vi "convertFromFPGA.vi"(0 "Modbus in":refnum<class "Modbus.lvclass">, 5 "Data":u16[](array[numeric]), 7 "StartIndex":i32, 9 "StopIndex":i32, 11 "error in (no error)":errorcluster, 12 "Timestamp":u64) -> (4 "Modbus out":refnum<class "Modbus.lvclass">, 6 "RxFrame":T1 {"Data" format="%02x"}, 15 "error out":errorcluster)   [LabVIEW 2016, in "RTModbusFPGA.lvlib" / "Modbus.lvclass"]
uses:
  Modbus.lvclass
  DataTypes/RxFrame.ctl
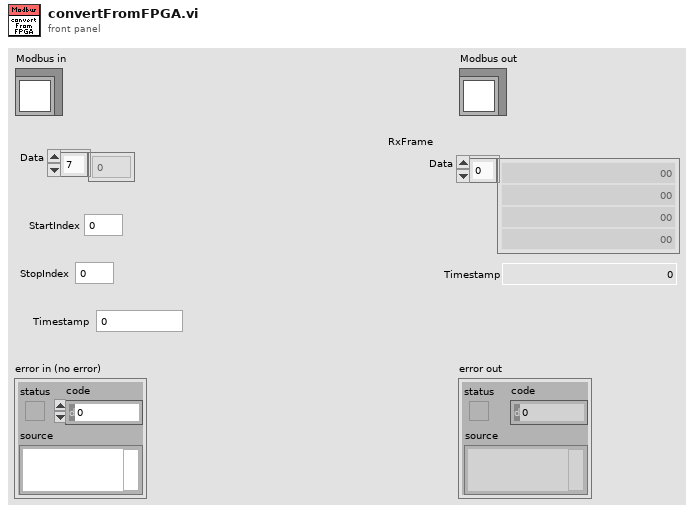
[diagram p1: front panel]
types:
  T1 = typedef "RxFrame.ctl" = cluster{"Data":u8[], "Timestamp":u64}
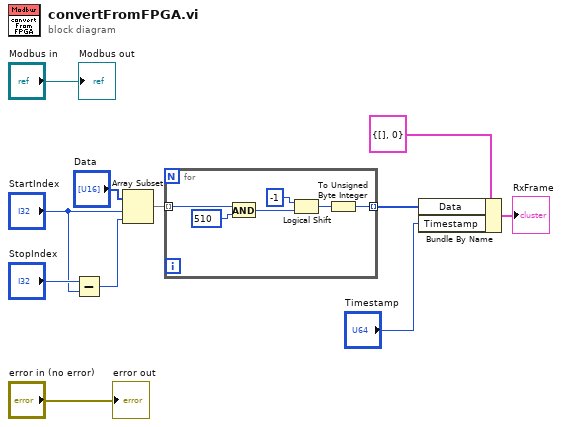
[diagram p0: block diagram]
diagram:
  n1 = Subtract(x="StopIndex", y="StartIndex") -> (x-y=w8:i32)
  n2 = Array Subset(array="Data", index="StartIndex", length=w8) -> (w7:u16[])
  n3 = for {
    tunnel: w7 -> [w12] mode=indexing
    tunnel: [w13] -> w2 mode=indexing
    n4 = And(x=w12, y=u16 510) -> (x .and. y?=w15:u16)
    n5 = Logical Shift(y=i16 -1, x=w15) -> (x << y=w14:u16)
    n6 = To Unsigned Byte Integer(number=w14) -> (unsigned 8bit integer=w13:u8)
  }
  n7 = Bundle By Name(cluster=T1 {"Data"=[], "Timestamp"=0} ("RxFrame"), "Data"=w2, "Timestamp"="Timestamp") -> (→"RxFrame":T1)
  "error out" <- "error in (no error)"
  "Modbus out" <- "Modbus in"
